vi "Begin.vi"(8 "error in":errorcluster) -> (0 "error out":errorcluster)   [LabVIEW 2023]
doc: "Called before other user functions, this VI is expected to open initial I/O refnums, load in file data, and do all program initialization. Notice that the <B>error out</B> terminal is simply used for data flow. Wiring it to other structures or subVIs ensures that this VI runs first."
uses:
  <vilib>/Rock Robotics/WPI/DriverStation/WPI_DriverStationRobotMode2.ctl
  <vilib>/Rock Robotics/WPI/Joystick/WPI_JoystickDeviceEnum.ctl
  <vilib>/Rock Robotics/SystemInterfaces/DIO/FPGA_DIOPWMChannel.ctl
  Robot Global Data.vi
  <vilib>/Rock Robotics/Network Tables/NT Write String Array.vi
  <vilib>/Rock Robotics/Network Tables/NT Write Boolean.vi
  <vilib>/Rock Robotics/WPI/MotorControl/WPI_MotorControlOpen SPARK_MAX.vi
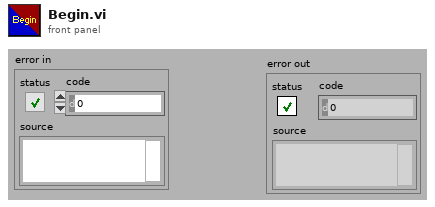
[diagram p1: front panel]
types:
  T1 = typedef "FPGA_DIOPWMChannel.ctl" = enum8{"PWM 0", "PWM 1", "PWM 2", "PWM 3", "PWM 4", "PWM 5", "PWM 6", "PWM 7", "PWM 8", "PWM 9", "PWM MXP 0", "PWM MXP 1", "PWM MXP 2", "PWM MXP 3", "PWM MXP 4", "PWM MXP 5", "PWM MXP 6", "PWM MXP 7", "PWM MXP 8", "PWM MXP 9", "Invalid"}
  T2 = typedef "WPI_JoystickDeviceEnum.ctl" = enum16{"USB 0", "USB 1", "USB 2", "USB 3", "USB 4", "USB 5"}
  T3 = typedef "WPI_DriverStationRobotMode2.ctl" = enum16{"Autonomous Disabled", "Autonomous Enabled", "Teleop Disabled", "Teleop Enabled", "Disconnected", "Finish", "Test Disabled", "Test Enabled", "Emergency Stopped"}
  T4 = typedef "CTRE_PigeonIMU_DeviceRef.ctl" = cluster{"DeviceStatus":errorcluster, "Device Number":u8, "Type":T5, "Device ID":u32, "Handle":u64, "UsageFrame":u32, "Library Path":path}
  T5 = typedef "CTRE_PigeonIMU_ConnectionType.ctl" = u32
  T6 = typedef "WPI_JoystickDevRef.ctl" = cluster{"Device":T2}
  T7 = typedef "WPI_MotorControlDeviceRef.ctl" = cluster{"DeviceStatus":errorcluster, "Type":T8, "PWM":cluster{"PWM Channel":T1, "DeadBand":T9}, "CAN":cluster{"Device Number":u8, "SetOutput VI Ref":variant, "GetOutput VI Ref":variant, "Enable VI Ref":variant, "Disable VI Ref":variant, "Data":variant}, "Invert":bool, "DIO PWM":cluster{"PWM \"Enable\" Channel":T1, "DIOChannel":T10, "PWM Rate":dbl}}
  T8 = typedef "WPI_MotorControlType.ctl" = enum16{"PWM", "CAN", "DIO PWM"}
  T9 = typedef "WPI_PWMDeadband.ctl" = cluster{"Name":string, "maxPositivePwm":i32, "minPositivePwm":i32, "centerPwm":i32, "maxNegativePwm":i32, "minNegativePwm":i32, "angularRange":u16}
  T10 = typedef "FPGA_DIOChannel.ctl" = enum8{"DIO 0", "DIO 1", "DIO 2", "DIO 3", "DIO 4", "DIO 5", "DIO 6", "DIO 7", "DIO 8", "DIO 9", "DIO MXP 0", "DIO MXP 1", "DIO MXP 2", "DIO MXP 3", "DIO MXP 4", "DIO MXP 5", "DIO MXP 6", "DIO MXP 7", "DIO MXP 8", "DIO MXP 9", "DIO MXP 10", "DIO MXP 11", "DIO MXP 12", "DIO MXP 13", "DIO MXP 14", "DIO MXP 15", "SPI Port CS1", "SPI Port CS2", "SPI Port CS3", "SPI Port MISO", "SPI Port MOSI", "Invalid"}
  T11 = typedef "CTRE_Phoenix_CANcoder_DeviceRef.ctl" = cluster{"DeviceStatus":errorcluster, "Device Number":u8, "Handle":u64, "UsageFrame":u32, "Library Path":path}
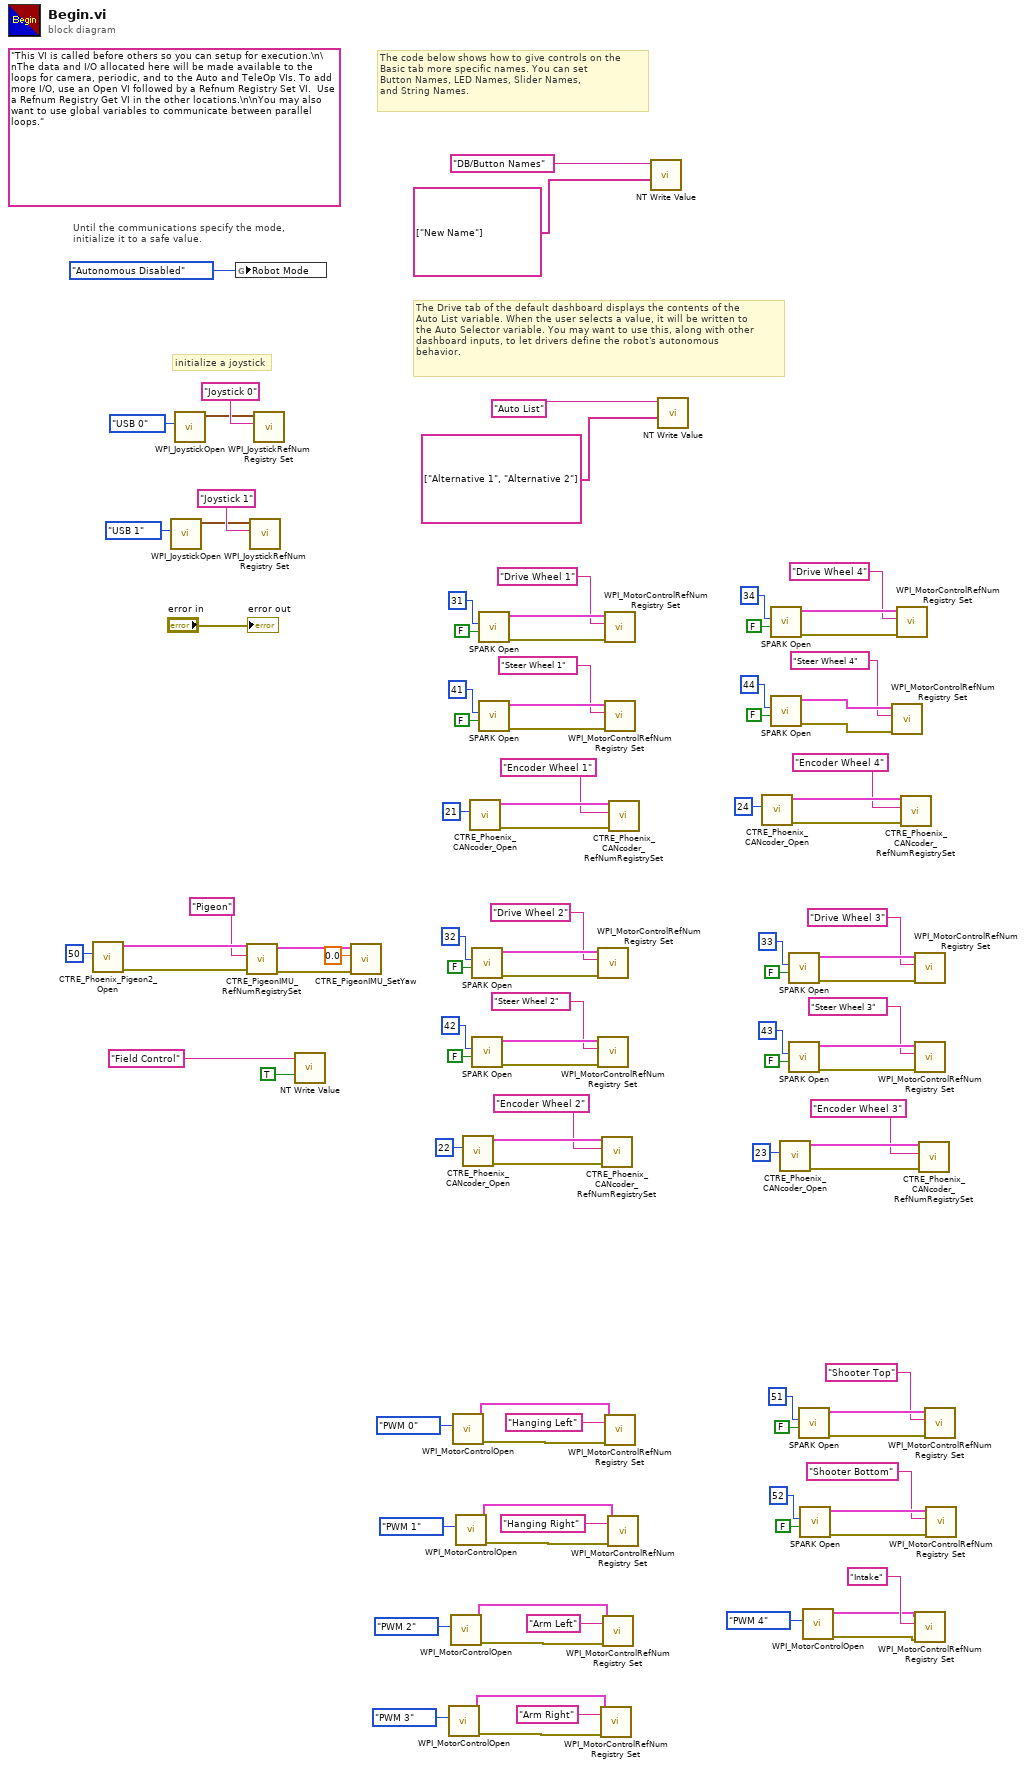
[diagram p0: block diagram]
diagram:
  (unwired) "This VI is called before others so you can setup for execution.\n\nThe data and I/O allocated here will be made available to the loops for camera, periodic, and to the Auto and TeleOp VIs. To add more I/O, use an Open VI followed by a Refnum Registry Set VI.  Use a Refnum Registry Get VI in the other locations.\n\nYou may also want to use global variables to communicate between parallel loops."
  # "The Drive tab of the default dashboard displays the contents of the\nAuto List variable. When the user selects a value, it will be written to\nthe Auto Selector variable. You may want to use this, along with other\ndashboard inputs, to let drivers define the robot's autonomous\nbehavior."
  # "The code below shows how to give controls on the\nBasic tab more specific names. You can set\nButton Names, LED Names, Slider Names,\nand String Names."
  # "initialize a joystick"
  # "Until the communications specify the mode,\ninitialize it to a safe value."
  n1 = call <vilib>:"CTRE_Phoenix_Pigeon2_Open.vi"("Device Number"=u8 50) -> ("error out"=w42:errorcluster, "PigeonIMUDevRef"=w41:T4)  [unwired: 9 in]
  n2 = call <vilib>:"WPI_JoystickOpen.vi"("JoystickDevice"=WPI_JoystickDeviceEnum."USB 1") -> ("JoystickDevRef"=w5:T6)  [unwired: 10 in]
  n3 = call <vilib>:"WPI_JoystickOpen.vi"("JoystickDevice"=WPI_JoystickDeviceEnum."USB 0") -> ("JoystickDevRef"=w105:T6)  [unwired: 10 in]
  n4 = global write "Robot Global Data.vi" "Robot Mode"(WPI_DriverStationRobotMode2."Autonomous Disabled" ("Robot Mode")) -> ()
  n5 = call <vilib>:"CTRE_PigeonIMU_RefNumRegistrySet.vi"("error in (no error)"=w42, "refnum name"="Pigeon", "PigeonIMUDevRef"=w41) -> ("error out"=w38:errorcluster, "PigeonIMUDevRef"=w37:T4)  [unwired: 7 in]
  n6 = call <vilib>:"WPI_JoystickRefNum Registry Set.vi"("refnum name"="Joystick 1", "JoystickDevRef"=w5) -> ()  [unwired: 8 in, 2 out]
  n7 = call <vilib>:"WPI_JoystickRefNum Registry Set.vi"("refnum name"="Joystick 0", "JoystickDevRef"=w105) -> ()  [unwired: 8 in, 2 out]
  n8 = call-poly <vilib>:"NT Write Value.vi"("value"=TRUE, "name"="Field Control") -> ()  [unwired: 9 in, 1 out]
  n9 = call <vilib>:"CTRE_PigeonIMU_SetYaw.vi"("error in (no error)"=w38, "Value"=0.0, "PigeonIMUDevRef"=w37) -> ()  [unwired: 7 in, 2 out]
  n10 = call-poly <vilib>:"WPI_MotorControlOpen.vi"("PWM Channel"=FPGA_DIOPWMChannel."PWM 3") -> ("error out"=w20:errorcluster, "MotorControlDeviceRef"=w19:T7)  [unwired: 9 in]
  n11 = call-poly <vilib>:"WPI_MotorControlOpen.vi"("PWM Channel"=FPGA_DIOPWMChannel."PWM 2") -> ("error out"=w24:errorcluster, "MotorControlDeviceRef"=w23:T7)  [unwired: 9 in]
  n12 = call-poly <vilib>:"WPI_MotorControlOpen.vi"("PWM Channel"=FPGA_DIOPWMChannel."PWM 0") -> ("error out"=w32:errorcluster, "MotorControlDeviceRef"=w31:T7)  [unwired: 9 in]
  n13 = call-poly <vilib>:"WPI_MotorControlOpen.vi"("PWM Channel"=FPGA_DIOPWMChannel."PWM 1") -> ("error out"=w28:errorcluster, "MotorControlDeviceRef"=w27:T7)  [unwired: 9 in]
  n14 = call <vilib>:"CTRE_Phoenix_CANcoder_Open.vi"("Device Number"=u8 22) -> ("error out"=w72:errorcluster, "CTRE_CANcoder_DeviceRef"=w73:T11)  [unwired: 9 in]
  n15 = call <vilib>:"CTRE_Phoenix_CANcoder_Open.vi"("Device Number"=u8 21) -> ("error out"=w86:errorcluster, "CTRE_CANcoder_DeviceRef"=w87:T11)  [unwired: 9 in]
  n16 = call <vilib>:"SPARK Open.vi"("Invert"=FALSE, "Device Number"=u8 32) -> ("error out"=w84:errorcluster, "MotorControlDeviceRef"=w83:T7)  [unwired: 8 in]
  n17 = call <vilib>:"SPARK Open.vi"("Invert"=FALSE, "Device Number"=u8 42) -> ("error out"=w79:errorcluster, "MotorControlDeviceRef"=w78:T7)  [unwired: 8 in]
  n18 = call <vilib>:"SPARK Open.vi"("Invert"=FALSE, "Device Number"=u8 31) -> ("error out"=w98:errorcluster, "MotorControlDeviceRef"=w97:T7)  [unwired: 8 in]
  n19 = call <vilib>:"SPARK Open.vi"("Invert"=FALSE, "Device Number"=u8 41) -> ("error out"=w93:errorcluster, "MotorControlDeviceRef"=w92:T7)  [unwired: 8 in]
  n20 = call <vilib>:"WPI_MotorControlRefNum Registry Set.vi"("error in (no error)"=w84, "refnum name"="Drive Wheel 2", "MotorControlDevRef"=w83) -> ()  [unwired: 7 in, 2 out]
  n21 = call <vilib>:"WPI_MotorControlRefNum Registry Set.vi"("error in (no error)"=w79, "refnum name"="Steer Wheel 2", "MotorControlDevRef"=w78) -> ()  [unwired: 7 in, 2 out]
  n22 = call <vilib>:"WPI_MotorControlRefNum Registry Set.vi"("error in (no error)"=w20, "refnum name"="Arm Right", "MotorControlDevRef"=w19) -> ()  [unwired: 7 in, 2 out]
  n23 = call <vilib>:"CTRE_Phoenix_CANcoder_RefNumRegistrySet.vi"("error in (no error)"=w72, "refnum name"="Encoder Wheel 2", "CTRE_CANcoder_DeviceRef"=w73) -> ()  [unwired: 7 in, 2 out]
  n24 = call <vilib>:"WPI_MotorControlRefNum Registry Set.vi"("error in (no error)"=w24, "refnum name"="Arm Left", "MotorControlDevRef"=w23) -> ()  [unwired: 7 in, 2 out]
  n25 = call <vilib>:"WPI_MotorControlRefNum Registry Set.vi"("error in (no error)"=w98, "refnum name"="Drive Wheel 1", "MotorControlDevRef"=w97) -> ()  [unwired: 7 in, 2 out]
  n26 = call <vilib>:"WPI_MotorControlRefNum Registry Set.vi"("error in (no error)"=w93, "refnum name"="Steer Wheel 1", "MotorControlDevRef"=w92) -> ()  [unwired: 7 in, 2 out]
  n27 = call <vilib>:"WPI_MotorControlRefNum Registry Set.vi"("error in (no error)"=w32, "refnum name"="Hanging Left", "MotorControlDevRef"=w31) -> ()  [unwired: 7 in, 2 out]
  n28 = call <vilib>:"WPI_MotorControlRefNum Registry Set.vi"("error in (no error)"=w28, "refnum name"="Hanging Right", "MotorControlDevRef"=w27) -> ()  [unwired: 7 in, 2 out]
  n29 = call <vilib>:"CTRE_Phoenix_CANcoder_RefNumRegistrySet.vi"("error in (no error)"=w86, "refnum name"="Encoder Wheel 1", "CTRE_CANcoder_DeviceRef"=w87) -> ()  [unwired: 7 in, 2 out]
  n30 = call-poly <vilib>:"NT Write Value.vi"("value"=string[] ["New Name"], "name"="DB/Button Names" ("Name")) -> ()  [unwired: 9 in, 1 out]
  n31 = call-poly <vilib>:"NT Write Value.vi"("value"=string[] ["Alternative 1", "Alternative 2"] ("String Array"), "name"="Auto List" ("Name")) -> ()  [unwired: 9 in, 1 out]
  n32 = call <vilib>:"CTRE_Phoenix_CANcoder_Open.vi"("Device Number"=u8 24) -> ("error out"=w44:errorcluster, "CTRE_CANcoder_DeviceRef"=w45:T11)  [unwired: 9 in]
  n33 = call <vilib>:"SPARK Open.vi"("Invert"=FALSE, "Device Number"=u8 34) -> ("error out"=w56:errorcluster, "MotorControlDeviceRef"=w55:T7)  [unwired: 8 in]
  n34 = call <vilib>:"SPARK Open.vi"("Invert"=FALSE, "Device Number"=u8 44) -> ("error out"=w51:errorcluster, "MotorControlDeviceRef"=w50:T7)  [unwired: 8 in]
  n35 = call <vilib>:"CTRE_Phoenix_CANcoder_Open.vi"("Device Number"=u8 23) -> ("error out"=w58:errorcluster, "CTRE_CANcoder_DeviceRef"=w59:T11)  [unwired: 9 in]
  n36 = call <vilib>:"SPARK Open.vi"("Invert"=FALSE, "Device Number"=u8 33) -> ("error out"=w70:errorcluster, "MotorControlDeviceRef"=w69:T7)  [unwired: 8 in]
  n37 = call <vilib>:"SPARK Open.vi"("Invert"=FALSE, "Device Number"=u8 43) -> ("error out"=w65:errorcluster, "MotorControlDeviceRef"=w64:T7)  [unwired: 8 in]
  n38 = call <vilib>:"SPARK Open.vi"("Invert"=FALSE, "Device Number"=u8 51) -> ("error out"=w17:errorcluster, "MotorControlDeviceRef"=w16:T7)  [unwired: 8 in]
  n39 = call <vilib>:"SPARK Open.vi"("Invert"=FALSE, "Device Number"=u8 52) -> ("error out"=w12:errorcluster, "MotorControlDeviceRef"=w11:T7)  [unwired: 8 in]
  n40 = call-poly <vilib>:"WPI_MotorControlOpen.vi"("PWM Channel"=FPGA_DIOPWMChannel."PWM 4") -> ("error out"=w1:errorcluster, "MotorControlDeviceRef"=w2:T7)  [unwired: 9 in]
  n41 = call <vilib>:"WPI_MotorControlRefNum Registry Set.vi"("error in (no error)"=w51, "refnum name"="Steer Wheel 4", "MotorControlDevRef"=w50) -> ()  [unwired: 7 in, 2 out]
  n42 = call <vilib>:"WPI_MotorControlRefNum Registry Set.vi"("error in (no error)"=w56, "refnum name"="Drive Wheel 4", "MotorControlDevRef"=w55) -> ()  [unwired: 7 in, 2 out]
  n43 = call <vilib>:"CTRE_Phoenix_CANcoder_RefNumRegistrySet.vi"("error in (no error)"=w44, "refnum name"="Encoder Wheel 4", "CTRE_CANcoder_DeviceRef"=w45) -> ()  [unwired: 7 in, 2 out]
  n44 = call <vilib>:"WPI_MotorControlRefNum Registry Set.vi"("error in (no error)"=w70, "refnum name"="Drive Wheel 3", "MotorControlDevRef"=w69) -> ()  [unwired: 7 in, 2 out]
  n45 = call <vilib>:"WPI_MotorControlRefNum Registry Set.vi"("error in (no error)"=w65, "refnum name"="Steer Wheel 3", "MotorControlDevRef"=w64) -> ()  [unwired: 7 in, 2 out]
  n46 = call <vilib>:"WPI_MotorControlRefNum Registry Set.vi"("error in (no error)"=w1, "refnum name"="Intake", "MotorControlDevRef"=w2) -> ()  [unwired: 7 in, 2 out]
  n47 = call <vilib>:"CTRE_Phoenix_CANcoder_RefNumRegistrySet.vi"("error in (no error)"=w58, "refnum name"="Encoder Wheel 3", "CTRE_CANcoder_DeviceRef"=w59) -> ()  [unwired: 7 in, 2 out]
  n48 = call <vilib>:"WPI_MotorControlRefNum Registry Set.vi"("error in (no error)"=w17, "refnum name"="Shooter Top", "MotorControlDevRef"=w16) -> ()  [unwired: 7 in, 2 out]
  n49 = call <vilib>:"WPI_MotorControlRefNum Registry Set.vi"("error in (no error)"=w12, "refnum name"="Shooter Bottom", "MotorControlDevRef"=w11) -> ()  [unwired: 7 in, 2 out]
  "error out" <- "error in"
